vi "Move rel mMc.vi"(0 "position incr":dbl, 1 "Port":T1={"P type"=0, "reference"="", " Terminator "="\r\n", "Timeout"=300} {"Timeout" step=10; "P type" items=["none", "RS-232C"]}, 3 "error in (no error)":errorcluster, 4 "rev dir?":bool caption="pos      neg", 5 "Controller #":string) -> (9 "error out":errorcluster)   [LabVIEW 2015]
doc: "MVR 命令：相对位置移动"
panel:
  # "Move relative"
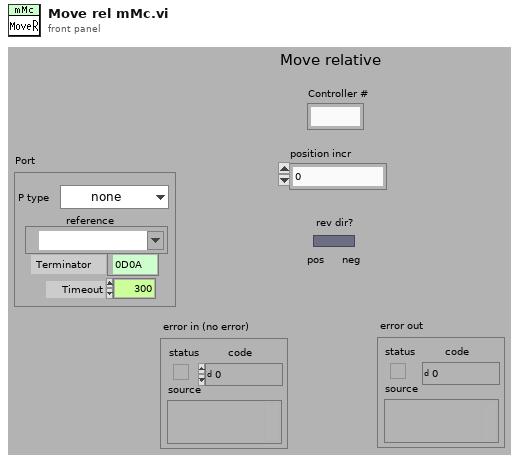
[diagram p1: front panel]
types:
  T1 = cluster{"P type":u16, "reference":refnum<visa-resource-name>, " Terminator ":string, "Timeout":i32}
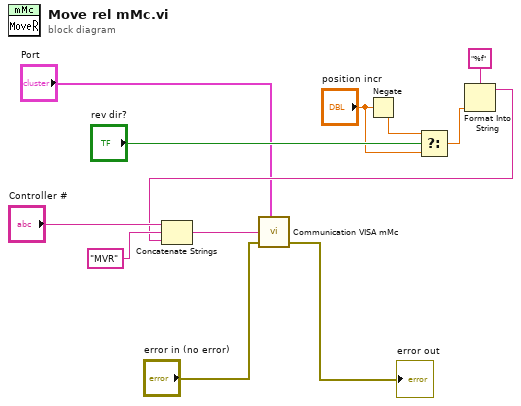
[diagram p0: block diagram]
diagram:
  n1 = Negate(x="position incr") -> (-x=w2:dbl)
  n2 = Select(t=w2, s="rev dir?", f="position incr") -> (s? t:f=w4:dbl)
  n3 = Format Into String(format string="%f", w4) -> (resulting string=w7:string)  [unwired: 2 in, 1 out]
  n4 = Concatenate Strings("Controller #", "MVR", w7) -> (w6:string)
  n5 = call <instrlib>:"Communication VISA mMc.vi"("Port"="Port", "Command"=w6, "error in (no error)"="error in (no error)") -> ("error out"=→"error out":errorcluster)  [unwired: 3 in, 3 out]
